vi "Create Channel from Xnet Signal.vi"(8 "error in (no error)":errorcluster, 10 "channel classification":T1, 11 "XNET Signal":refnum<k21>) -> (0 "error out":errorcluster, 2 "channel":refnum<class "TBM channel.lvclass">, 3 "XNET Signal 2":refnum<k21>)   [LabVIEW 2014, in "J1939 configuration.lvclass"]
uses:
  J1939 configuration.lvclass
  <vilib>/NI/Tag Bus Module Framework/channel/channel classification.ctl
  <vilib>/NI/Tag Bus Module Framework/channel/TBM channel.lvclass
  <resource>/objmgr/xnet.rc
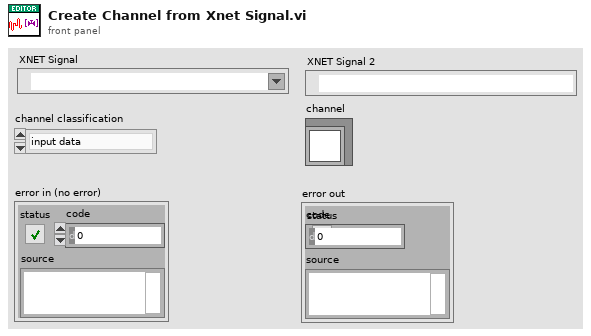
[diagram p1: front panel]
types:
  T1 = typedef "TBM channel.lvclass/channel classification.ctl" = enum16{"input data", "output data", "processing parameter", "processing result"}
  T2 = typedef "tag bus.lvlib/tag descriptor.lvclass/Data Type.ctl" = enum16{"Double", "Single", "I64", "I32", "I16", "I8", "U64", "U32", "U16", "U8", "Boolean", "String", "Array of Double", "Array of Single", "Array of I64", "Array of I32", "Array of I16", "Array of I8", "Array of U64", "Array of U32", "Array of U16", "Array of U8", "Array of Boolean", "Array of String"}
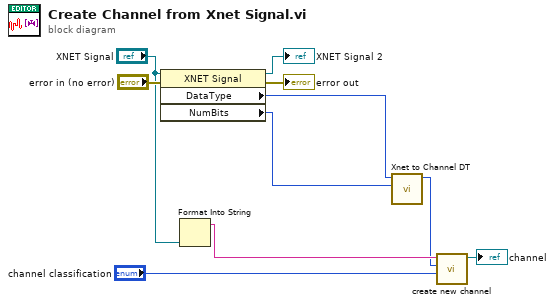
[diagram p0: block diagram]
diagram:
  n1 = property class="XNET Signal"(reference="XNET Signal", error in="error in (no error)") -> (reference out=→"XNET Signal 2":refnum<k21>, error out=→"error out":errorcluster, "DataType"=w9:u32, "NumBits"=w10:u32)
  n2 = Format Into String("XNET Signal") -> (resulting string=w4:string)  [unwired: 3 in, 1 out]
  n3 = call "Xnet to Channel DT.vi"("NumBits"=w10, "DataType"=w9) -> ("data type"=w3:T2)  [unwired: 9 in]
  n4 = call <vilib>:"create new channel.vi"("channel classification"="channel classification", "data type"=w3, "channel name"=w4) -> ("channel"=→"channel":refnum<class "TBM channel.lvclass">)  [unwired: 8 in]
